vi "NISE.Get Property DataType.vi"(0 "SLSC Interface in":refnum<class "SLSC Interface.lvclass">, 5 "property":refnum<k21>, 11 "error in (no error)":errorcluster) -> (4 "SLSC Interface out":refnum<class "SLSC Interface.lvclass">, 6 "property out":refnum<k21>, 10 "Prop.DataType":i32(ring) items=["None", "Bool", "DBL", "I32", "I64", "String", "U32", "U64", "1D Bool", "1D DBL", "1D I32", "1D I64", "1D String", "1D U32", "1D U64"], 15 "error out":errorcluster)   [LabVIEW 2016, in "SLSC Interface.lvclass"]
uses:
  SLSC Interface.lvclass
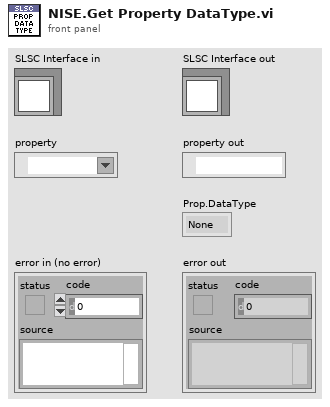
[diagram p1: front panel]
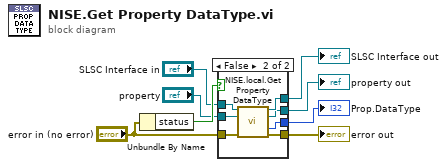
[diagram p0: block diagram]
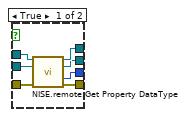
[diagram p2: hidden frame]
diagram:
  n1 = Unbundle By Name("error in (no error)") -> ("status"=w8:bool)
  n2 = case shown="False" w8 {
    tunnel: "SLSC Interface in" -> [w15 w22]
    tunnel: [w14 w21] -> w6
    tunnel: "property" -> [w13 w20]
    tunnel: [w12 w19] -> w4
    tunnel: [w11 w18] -> w3
    tunnel: "error in (no error)" -> [w10 w17]
    tunnel: [w9 w16] -> w1
    frame True {
      n3 = call "NISE.remote.Get Property DataType.vi"("SLSC Remote in"=w15, "property"=w13, "error in (no error)"=w10) -> ("SLSC Remote out"=w14:refnum<class "SLSC Interface.lvclass">, "property out"=w12:refnum<k21>, "Prop.DataType"=w11:i32, "error out"=w9:errorcluster)  [unwired: 9 in]
    }
    frame False {
      n4 = call "NISE.local.Get Property DataType.vi"("SLSC Local in"=w22, "property"=w20, "error in (no error)"=w17) -> ("SLSC Local out"=w21:refnum<class "SLSC Interface.lvclass">, "property out"=w19:refnum<k21>, "Prop.DataType"=w18:i32, "error out"=w16:errorcluster)  [unwired: 9 in]
    }
  }
  "error out" <- w1
  "SLSC Interface out" <- w6
  "property out" <- w4
  "Prop.DataType" <- w3
